vi "Enqueue ActorRef.vi"(8 "error in (no error)":errorcluster, 9 "UIRef":refnum<class "Message Enqueuer.lvclass">, 11 "MainUI Panel in":refnum<class "MainUI Panel.lvclass">) -> (0 "error out":errorcluster, 3 "MainUI Panel out":refnum<class "MainUI Panel.lvclass">)   [LabVIEW 2019, in "MainUI.lvlib" / "MainUI Panel.lvlib" / "MainUI Panel.lvclass"]
uses:
  MainUI Panel.lvclass
  ModuleAbstract/ModuleAbstract.lvclass
  <vilib>/ActorFramework/Message Enqueuer/Message Enqueuer.lvclass
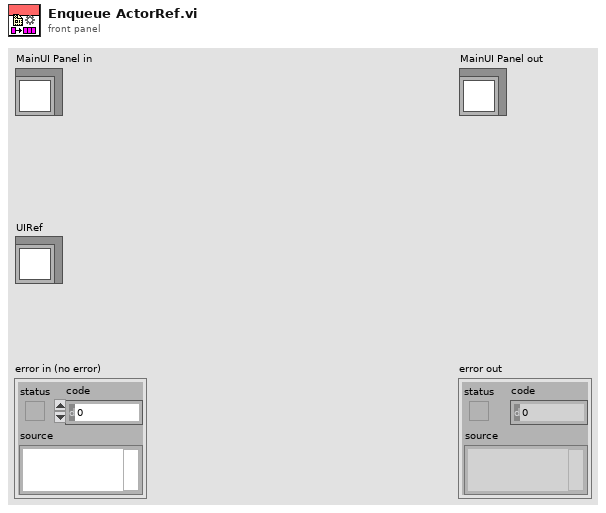
[diagram p1: front panel]
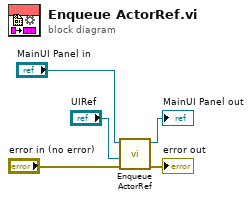
[diagram p0: block diagram]
diagram:
  n1 = call-parent "Enqueue ActorRef.vi"("error in (no error)"="error in (no error)", "UIRef"="UIRef", "ModuleAbstract in"="MainUI Panel in") -> ("error out"=→"error out":errorcluster, "ModuleAbstract out"=→"MainUI Panel out":refnum<class "MainUI Panel.lvclass">)  [unwired: 7 in]
